vi "Main.vi"() -> ()   [LabVIEW 2016]
doc: "The main Unicorn VI running all processes on the roboRIO.\nWhen running, a FPGA bitfile is read so the DIO ports will be dedicated to the FPGA."
uses:
  GlobalVI.vi
  builds/UnicornMain/UnicornRIO1/ROS for LabVIEW/home/lvuser/natinst/bin/user.lib/ROS for LabVIEW Software/ROS/Code/_ROSDefinition.vi
  <vilib>/myRIO/Express VI/Onboard Devices/LED/LED Express VI.xnode
  <vilib>/myRIO/Instrument Drivers/Onboard IO/DIO/vis/Write.vi
  <vilib>/myRIO/Instrument Drivers/Onboard IO/DIO/DIO.lvlib
  <vilib>/myRIO/Common/Instrument Driver Framework/myRIO v1.0/DIO/typedefs/DIO Channels Enum.ctl
  <vilib>/myRIO/Common/Instrument Driver Framework/myRIO v1.0/DIO/typedefs/DIO Channels List.ctl
  <vilib>/myRIO/Common/Instrument Driver Framework/Utilities/typedefs/Generic FPGA Reference.ctl
  <vilib>/myRIO/Common/Instrument Driver Framework/Utilities/typedefs/myRIO v1.0 Reference.ctl
  <vilib>/myRIO/Common/Instrument Driver Framework/Utilities/typedefs/Hardware Version Enum.ctl
  <vilib>/myRIO/Common/Instrument Driver Framework/Utilities/typedefs/myRIO Generic Hardware Reference.ctl
  <vilib>/myRIO/Instrument Drivers/Onboard IO/DIO/typedefs/DIO Reference.ctl
  <vilib>/myRIO/Instrument Drivers/Onboard IO/DIO/vis/myRIO DIO Open.xnode
  <vilib>/myRIO/Common/Instrument Driver Framework/Utilities/vis/Is FPGA Ref Available.vi
  <vilib>/myRIO/Common/Instrument Driver Framework/roboRIO v1.0/DIO/vis/roboRIO v1.0 Open DIO.vi
  <vilib>/userdefined/High Color/nirio_resource_hc.ctl
  <vilib>/rvi/interface/nirviCloseFPGA/nirviCloseFPGA.xnode
  <vilib>/FPGAPlugInAG/Dynamic/niLvFpga_Close_Dynamic.vi
  <vilib>/rvi/interface/nirviMethod/nirviMethod.xnode
  <vilib>/FPGAPlugInAG/Dynamic/niLvFpga_Reset_Dynamic.vi
  <vilib>/FPGAPlugInAG/Dynamic/niLvFpga_Run_Dynamic.vi
  <vilib>/myRIO/Instrument Drivers/Utilities/Utilities.lvlib
  <vilib>/FPGAPlugInAG/Dynamic/niLvFpga_StartFifo_Dynamic.vi
  <vilib>/rvi/errors/niLvFpgaMergeErrorWithErrorCode.vi
  <vilib>/myRIO/Express VI/Onboard Devices/Button/Button Express VI.xnode
  <vilib>/myRIO/Instrument Drivers/Onboard IO/DIO/vis/Read.vi
  <vilib>/rvi/interface/nirviOpenFPGA/nirviOpenFPGA.xnode
  FPGA/FPGA Bitfiles/UnicornMain_FPGATarget_MainFPGAcode_pijQzTnE6Wg.lvbitx
  <vilib>/FPGAPlugInAG/roboRIO/niLvFpga_Open_roboRIO.vi
  <vilib>/rvi/interface/common/dynamic/niFpgaDynamicAddResources.vi
panel:
  out "timeout":u32
  out "StartTime":u32
  out "FPGA REF Error out":errorcluster
  out "currentDirection":i32
  out "Sytem Online":bool
  out "Emergency STOP":bool
  out "runLidarBack":bool
  out "z":dbl
  out "y":dbl
  out "x":dbl
  out "runLiftStatemachine":bool
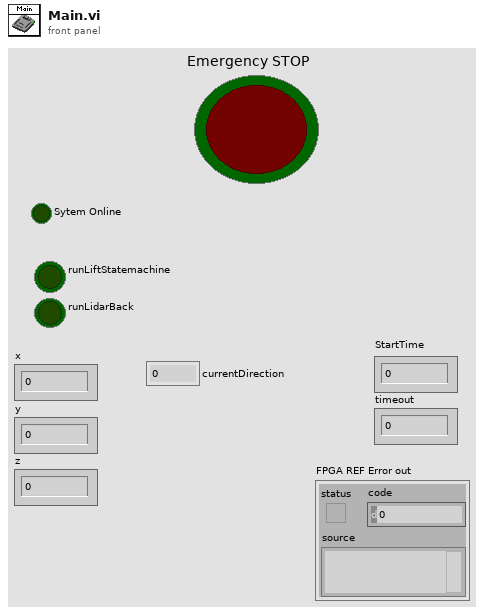
[diagram p1: front panel]
types:
  T1 = typedef "DIO.lvlib/DIO Reference.ctl" = cluster{"myRIO Reference":T2, "DIO Channels List":T6}
  T2 = typedef "myRIO Generic Hardware Reference.ctl" = cluster{"myRIO Model":T3, "myRIO Hardware Reference":T4}
  T3 = typedef "Hardware Version Enum.ctl" = enum16{"Unknown", "myRIO-1900", "myRIO-1950", "roboRIO", "NI ELVIS RIO CM"}
  T4 = typedef "myRIO v1.0 Reference.ctl" = cluster{"Generic FPGA Reference":T5, "Allow multiple opens":bool}
  T5 = typedef "Generic FPGA Reference.ctl" = refnum<k20>
  T6 = typedef "DIO Channels List.ctl" = T7[]
  T7 = typedef "DIO Channels Enum.ctl" = enum16{"Not Connected", "C/DIO0", "C/DIO1", "C/DIO2", "C/DIO3", "C/DIO4", "C/DIO5", "C/DIO6", "C/DIO7", "A/DIO0", "A/DIO1", "A/DIO2", "A/DIO3", "A/DIO4", "A/DIO5", "A/DIO6", "A/DIO7", "A/DIO8", "A/DIO9", "A/DIO10", "A/DIO11", "A/DIO12", "A/DIO13", "A/DIO14", "A/DIO15", "B/DIO0", "B/DIO1", "B/DIO2", "B/DIO3", "B/DIO4", "B/DIO5", "B/DIO6", "B/DIO7", "B/DIO8", "B/DIO9", "B/DIO10", "B/DIO11", "B/DIO12", "B/DIO13", "B/DIO14", "B/DIO15", "LED0", "LED1", "LED2", "LED3", "Button0", "DIO/DIO0", "DIO/DIO1", "DIO/DIO2", "DIO/DIO3", "DIO/DIO4", "DIO/DIO5", "DIO/DIO6", "DIO/DIO7", "DIO/DIO8", "DIO/DIO9", "SPI/CS0", "SPI/CS1", "SPI/CS2", "SPI/CS3", "LED RADIO (Green)", "LED RADIO (Red)", "LED COMM (Green)", "LED COMM (Red)", "LED MODE (Green)", "LED MODE (Red)"}
  T8 = typedef "nirio_resource_hc.ctl" = tag
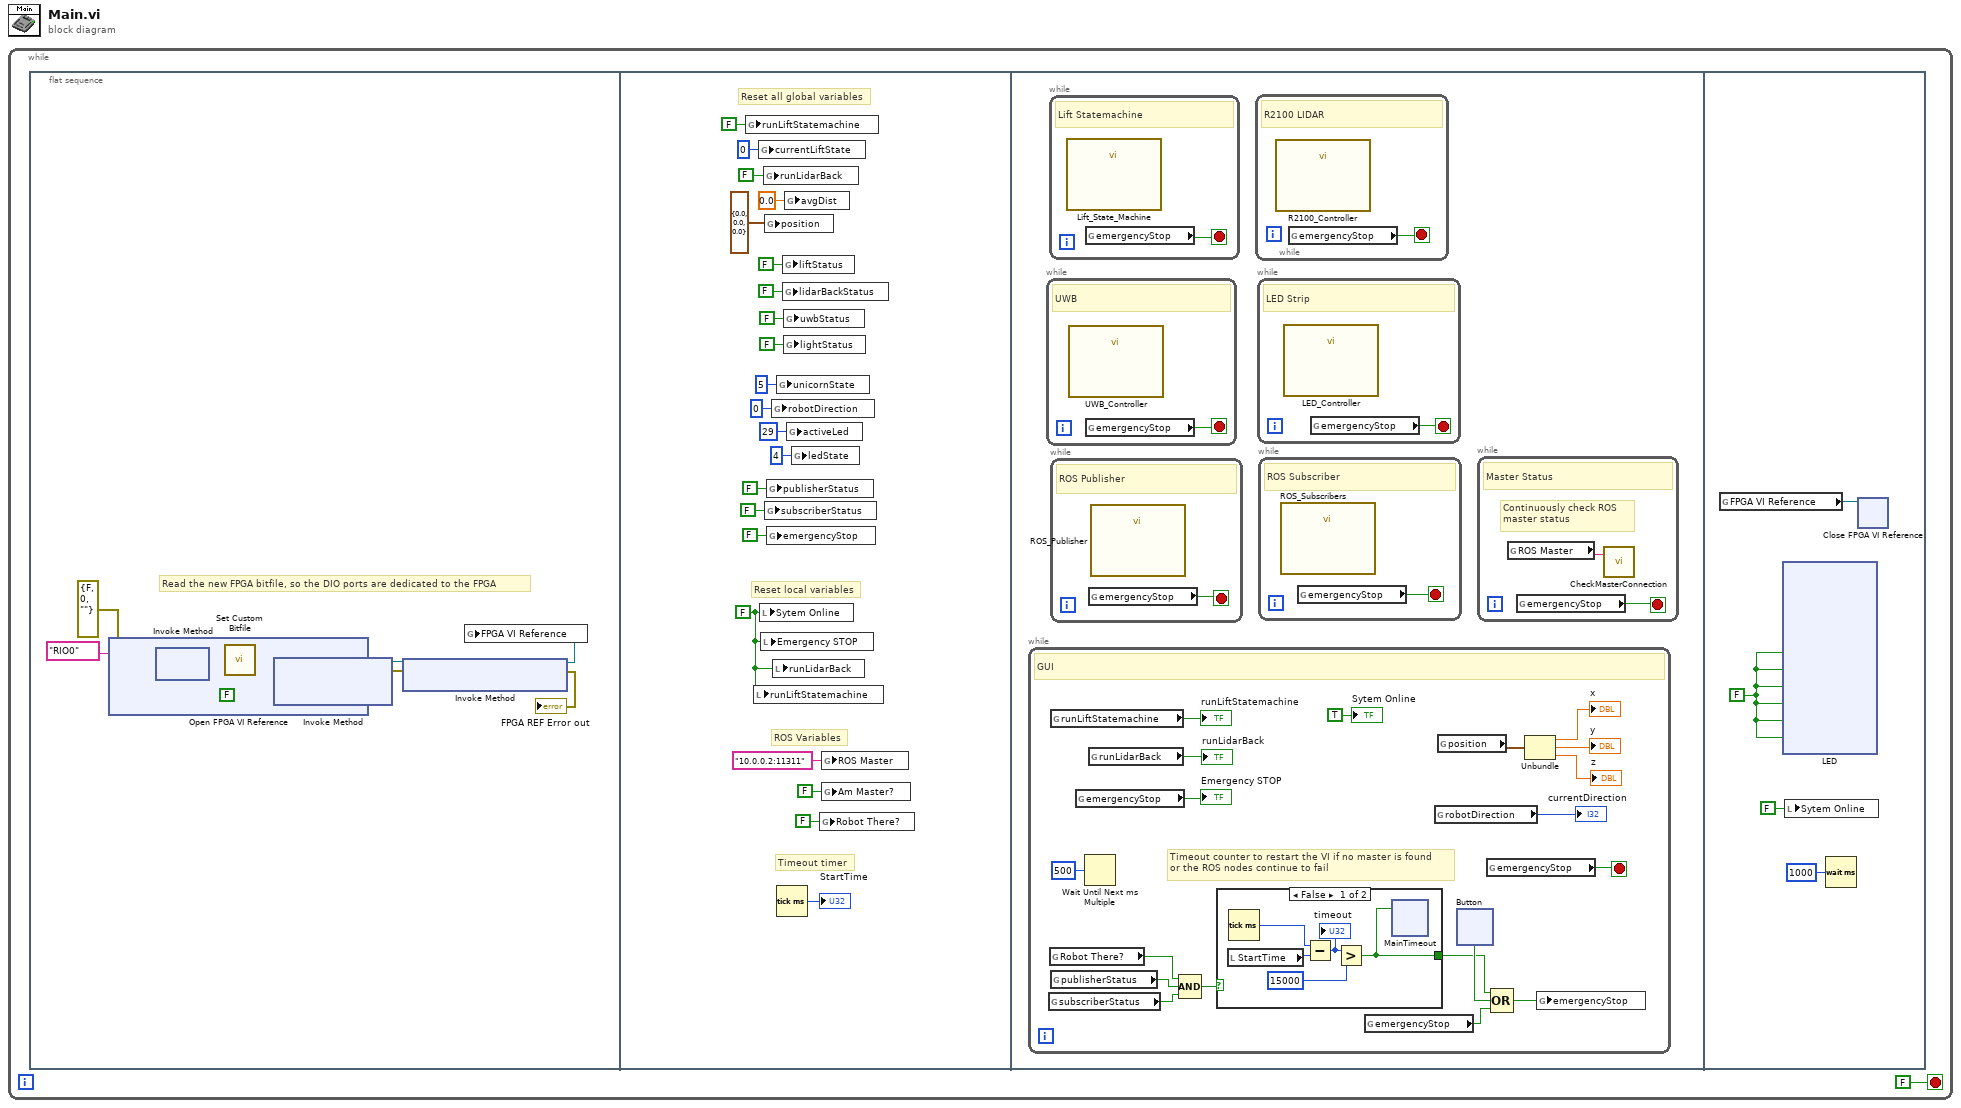
[diagram p0: block diagram]
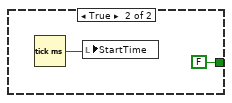
[diagram p2: hidden frame]
diagram:
  n1 = while {
    stop <- FALSE stop-if-true
    n2 = flat-sequence {
      frame #0 {
        # "Read the new FPGA bitfile, so the DIO ports are dedicated to the FPGA"
        n3 = xnode "Open FPGA VI Reference"("error in"=errorcluster {"status"=FALSE, "code"=0, "source"=""}, "resource name"=tag "RIO0") -> ("FPGA VI Reference Out"=w7:refnum<k20>, "error out"=w8:errorcluster)
        n4 = xnode "Invoke Method"("FPGA VI Reference In"=w7, "error in"=w8) -> ("FPGA VI Reference Out"=w11:refnum<k20>, "error out"=w10:errorcluster)
        n5 = call <vilib>:"Set Custom Bitfile.vi"("error in (no error)"=w10, "Custom FPGA Reference In"=w11) -> ("error out"=w12:errorcluster, "Custom FPGA Reference Out"=w13:refnum<k20>)  [unwired: 8 in]
        n6 = xnode "Invoke Method"("FPGA VI Reference In"=w13, "error in"=w12, "Wait Until Done (F)"=FALSE) -> ("FPGA VI Reference Out"=w5:refnum<k20>, "error out"=w4:errorcluster)
        n7 = xnode "Invoke Method"("FPGA VI Reference In"=w5, "error in"=w4) -> ("FPGA VI Reference Out"=w3:refnum<k20>, "error out"=→"FPGA REF Error out":errorcluster)
        n8 = global write "GlobalVI.vi" "FPGA VI Reference"(w3) -> ()
      }
      frame #1 {
        w27 = FALSE ("Sytem Online")
        # "Timeout timer"
        # "ROS Variables"
        # "Reset local variables"
        # "Reset all global variables"
        n9 = global write "GlobalVI.vi" "runLiftStatemachine"(FALSE ("runLiftStatemachine")) -> ()
        n10 = local write "runLiftStatemachine"(w27) -> ()
        n11 = global write "GlobalVI.vi" "currentLiftState"(0 ("currentLiftState")) -> ()
        n12 = local write "Sytem Online"(w27) -> ()
        n13 = local write "Emergency STOP"(w27) -> ()
        n14 = global write "GlobalVI.vi" "runLidarBack"(FALSE ("runLidarBack")) -> ()
        n15 = global write "GlobalVI.vi" "position"(cluster{"x":dbl, "y":dbl, "z":dbl} {"x"=0.0, "y"=0.0, "z"=0.0} ("position")) -> ()
        n16 = global write "GlobalVI.vi" "subscriberStatus"(FALSE ("subscriberStatus")) -> ()
        n17 = global write "GlobalVI.vi" "publisherStatus"(FALSE ("publisherStatus")) -> ()
        n18 = global write "GlobalVI.vi" "emergencyStop"(FALSE ("emergencyStop")) -> ()
        n19 = global write "GlobalVI.vi" "robotDirection"(0 ("robotDirection")) -> ()
        n20 = local write "runLidarBack"(w27) -> ()
        n21 = global write "GlobalVI.vi" "unicornState"(5 ("unicornState")) -> ()
        n22 = Tick Count (ms)() -> (millisecond timer value=→"StartTime":u32)
        n23 = global write "GlobalVI.vi" "liftStatus"(FALSE ("liftStatus")) -> ()
        n24 = global write "GlobalVI.vi" "lidarBackStatus"(FALSE ("lidarBackStatus")) -> ()
        n25 = global write "GlobalVI.vi" "uwbStatus"(FALSE ("uwbStatus")) -> ()
        n26 = global write "GlobalVI.vi" "lightStatus"(FALSE ("lightStatus")) -> ()
        n27 = global write "GlobalVI.vi" "avgDist"(sgl 0.0 ("avgDist")) -> ()
        n28 = global write "GlobalVI.vi" "activeLed"(29 ("activeLed")) -> ()
        n29 = global write "GlobalVI.vi" "ledState"(4 ("ledState")) -> ()
        n30 = global write "_ROSDefinition.vi" "Robot There?"(FALSE ("Robot There?")) -> ()
        n31 = global write "_ROSDefinition.vi" "ROS Master"("10.0.0.2:11311" ("ROS Master")) -> ()
        n32 = global write "_ROSDefinition.vi" "Am Master?"(FALSE ("Am Master?")) -> ()
      }
      frame #2 {
        n33 = while {
          stop <- w56 stop-if-true
          # "Timeout counter to restart the VI if no master is found\nor the ROS nodes continue to fail"
          # "GUI"
          n34 = global read "GlobalVI.vi" "subscriberStatus"() -> (w46:bool)
          n35 = global read "_ROSDefinition.vi" "Robot There?"() -> (w48:bool)
          n36 = global read "GlobalVI.vi" "runLiftStatemachine"() -> (→"runLiftStatemachine":bool)
          n37 = global read "GlobalVI.vi" "publisherStatus"() -> (w47:bool)
          n38 = global read "GlobalVI.vi" "emergencyStop"() -> (→"Emergency STOP":bool)
          n39 = Wait Until Next ms Multiple(millisecond multiple=u32 500) -> ()  [unwired: 1 out]
          n40 = global read "GlobalVI.vi" "runLidarBack"() -> (→"runLidarBack":bool)
          n41 = Compound Arithmetic op=AND(w48, w47, w46) -> (w45:bool)
          n42 = case shown="False" w45 {
            tunnel: [w62 FALSE] -> w49
            frame False {
              n43 = local read "StartTime"() -> (w66:u32)
              n44 = Tick Count (ms)() -> (millisecond timer value=w65:u32)
              n45 = Subtract(x=w65, y=w66) -> (x-y=w64:u32)
              "timeout" <- w64
              n46 = Greater?(x=w64, y=u32 15000) -> (0:w62:bool)
              n47 = xnode ("MainTimeout")("RADIO (Red)"=w62) -> ()  [unwired: 1 in, 1 out]
            }
            frame True {
              n48 = Tick Count (ms)() -> (millisecond timer value=w102:u32)
              n49 = local write "StartTime"(w102) -> ()
            }
          }
          n50 = global read "GlobalVI.vi" "emergencyStop"() -> (w43:bool)
          n51 = global read "GlobalVI.vi" "robotDirection"() -> (→"currentDirection":i32)
          n52 = global read "GlobalVI.vi" "position"() -> (w60:cluster{"x":dbl, "y":dbl, "z":dbl})
          n53 = xnode "Button"() -> ("Value"=w50:bool)  [unwired: 1 in, 1 out]
          n54 = global read "GlobalVI.vi" "emergencyStop"() -> (w56:bool)
          n55 = Compound Arithmetic op=OR(w49, w50, w43) -> (w44:bool)
          n56 = Unbundle(w60) -> ("x"=→"x":dbl, "y"=→"y":dbl, "z"=→"z":dbl)
          n57 = global write "GlobalVI.vi" "emergencyStop"(w44) -> ()
          "Sytem Online" <- TRUE ("Sytem Online")
        }
        n58 = while {
          stop <- w36 stop-if-true
          # "UWB"
          n59 = call "UWB_Controller.vi"() -> ()  [unwired: 12 in]
          n60 = global read "GlobalVI.vi" "emergencyStop"() -> (w36:bool)
        }
        n61 = while {
          stop <- w139 stop-if-true
          # "Lift Statemachine"
          n62 = call "Lift_State_Machine.vi"() -> ()  [unwired: 12 in]
          n63 = global read "GlobalVI.vi" "emergencyStop"() -> (w139:bool)
        }
        n64 = while {
          stop <- w40 stop-if-true
          # "ROS Publisher"
          n65 = global read "GlobalVI.vi" "emergencyStop"() -> (w40:bool)
          n66 = call "ROS_Publisher.vi"() -> ()  [unwired: 12 in]
        }
        n67 = while {
          stop <- w42 stop-if-true
          # "R2100 LIDAR"
          n68 = call "R2100_Controller.vi"() -> ()  [unwired: 11 in]
          n69 = global read "GlobalVI.vi" "emergencyStop"() -> (w42:bool)
        }
        n70 = while {
          stop <- w39 stop-if-true
          # "LED Strip"
          n71 = call "LED_Controller.vi"() -> ()  [unwired: 12 in]
          n72 = global read "GlobalVI.vi" "emergencyStop"() -> (w39:bool)
        }
        n73 = while {
          stop <- w41 stop-if-true
          # "ROS Subscriber"
          n74 = call "ROS_Subscribers.vi"() -> ()  [unwired: 12 in]
          n75 = global read "GlobalVI.vi" "emergencyStop"() -> (w41:bool)
        }
        n76 = while {
          stop <- w37 stop-if-true
          # "Continuously check ROS\nmaster status"
          # "Master Status"
          n77 = global read "_ROSDefinition.vi" "ROS Master"() -> (w38:string)
          n78 = global read "GlobalVI.vi" "emergencyStop"() -> (w37:bool)
          n79 = call "CheckMasterConnection.vi"("Master IP"=w38) -> ()  [unwired: 1 in, 2 out]
        }
      }
      frame #3 {
        w143 = FALSE
        n80 = global read "GlobalVI.vi" "FPGA VI Reference"() -> (w141:refnum<k20>)
        n81 = xnode "LED"("RADIO (Green)"=w143, "RADIO (Red)"=w143, "COMM (Green)"=w143, "COMM (Red)"=w143, "MODE (Green)"=w143, "MODE (Red)"=w143) -> ()  [unwired: 1 in, 1 out]
        n82 = local write "Sytem Online"(FALSE ("Sytem Online")) -> ()
        n83 = Wait (ms)(milliseconds to wait=u32 1000) -> ()  [unwired: 1 out]
        n84 = xnode "Close FPGA VI Reference"("FPGA VI Reference In"=w141) -> ()  [unwired: 1 in, 1 out]
      }
    }
  }
